vi "Grid Measurements Example - Topo & GridSpectr.vi"(6 "Internal use":string, 7 "Grid param":T1 {"height (m)" format="%#_6p"; "width (m)" format="%#_6p"; "center Y (m)" format="%#_6p"; "center X (m)" format="%#_6p"}, 8 "Error in (no error)":errorcluster, 9 "Points Y/Index Y":i32, 10 "Points X/Index X":i32, 11 "Method":enum16{"init", "run", "end"}(ring)) -> (0 "Error out":errorcluster)   [LabVIEW 2016]
doc: "Example of a measurement VI to be used in the \"Experiments on a Grid\" tool as external VI.\n\nThis example measure the topography and spectroscopy data. The spectroscopy measurements are taken on a subgrid. The data are saved to a sxm and a binary file.\n\n- Nanonis Programming Interface -"
uses:
  Nanonis Prog Interface.lvlib
  Instance           1 53Saved   Grid Measurements Example - Topo & GridSpectr .vi
panel:
  in  "Y subgrid spacing":u16=4
  in  "X subgrid spacing":u16=4
  # "Example of a measurement VI to be used in the \"Experiments on a Grid\" tool as external VI.\n\nThis example measure the topography and spectroscopy data. The spectroscopy measurements are taken on a subgrid. The data are saved to a sxm and a binary file.\n\nTo use it, set up the bias spectroscopy module to record the desired channels and set all other spectroscopy parameters. Then, set up the experiments on a grid module to use this VI as \"external VI\". On this VI's front panel, adjust the subgrid spacing.\n\n\"Experiments on a Grid\" will first (before starting the measurements) call the external VI with the \"init\" method, passing the grid resolution (Points X, Points Y) and the grid dimensions (Grid).\nThen, for the measurements, the external VI will be called with the \"run\" method, passing the current X and Y indices (Index X, Index Y).\nAfter the last measurement, the external VI will be called using the \"end\" method.\n\nSee diagram for more information about this example."
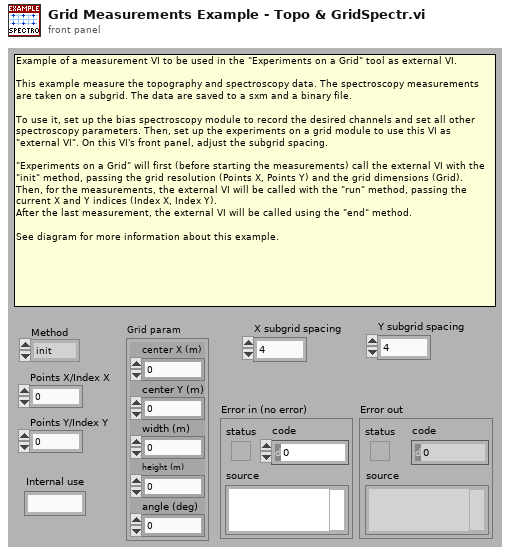
[diagram p1: front panel]
types:
  T1 = cluster{"center X (m)":sgl, "center Y (m)":sgl, "width (m)":sgl, "height (m)":sgl, "angle (deg)":sgl}
  T2 = cluster{"center X":sgl, "center Y":sgl, "angle":sgl, "width":sgl, "height":sgl, "# pixels":i32, "# lines":i32}
  T3 = cluster{"Name":string, "Calibration":sgl, "Offset":sgl, "Channel index":i32}[]
  T4 = cluster{"up/down":bool, "time/line":sgl, "start time":timestamp, "end time":timestamp}
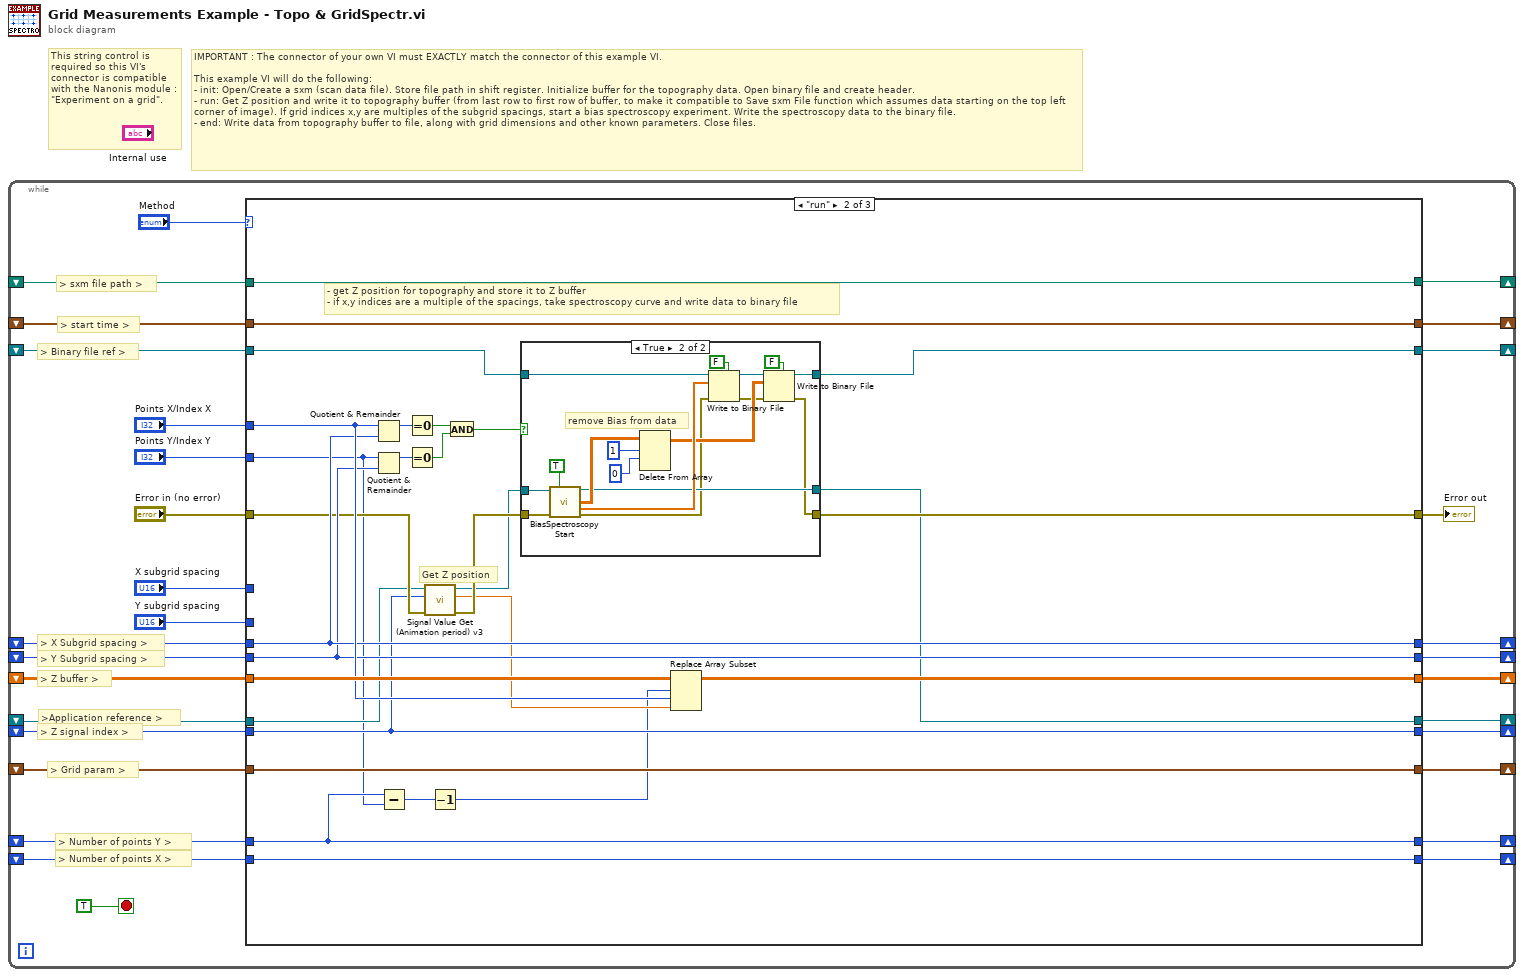
[diagram p0: block diagram]
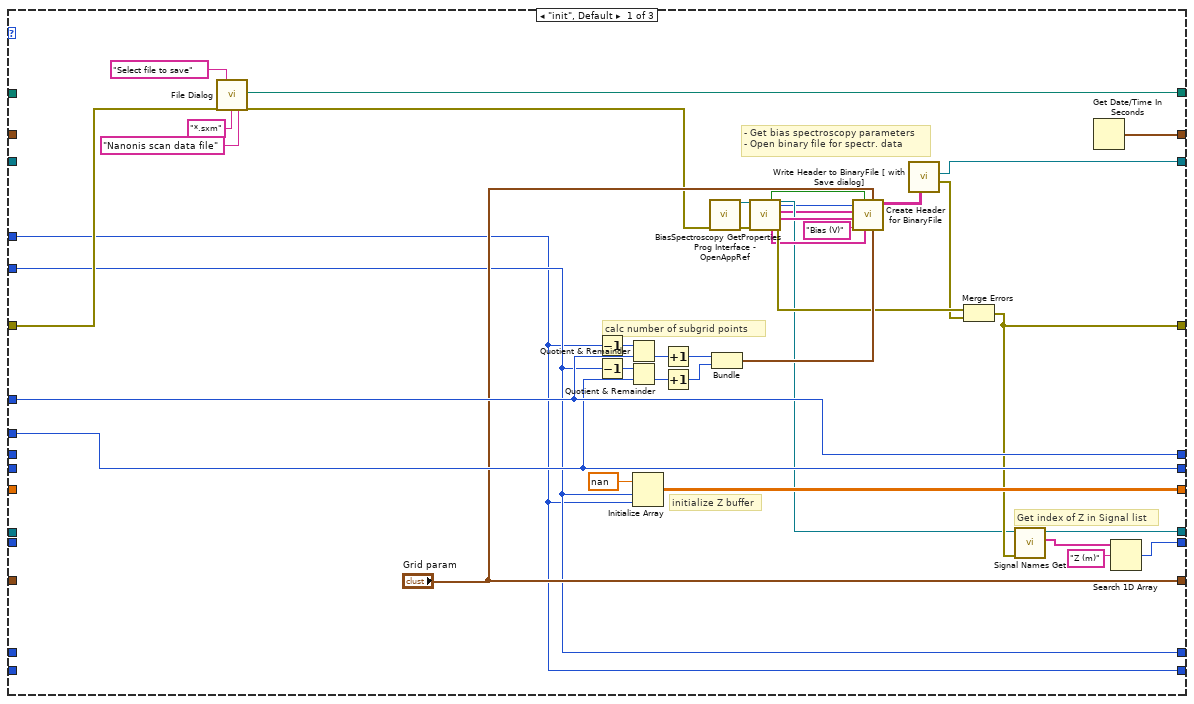
[diagram p2: hidden frame]
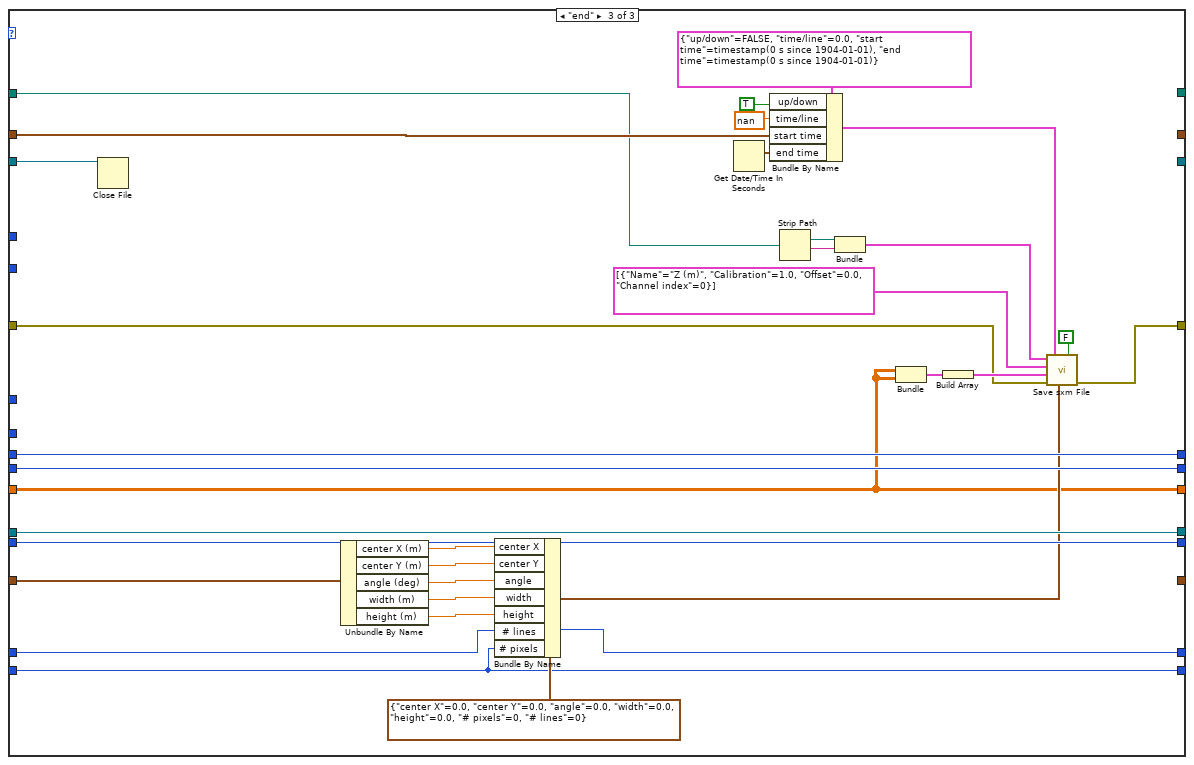
[diagram p4: hidden frame]
diagram:
  # "This string control is required so this VI's connector is compatible with the Nanonis module : \"Experiment on a grid\"."
  # "IMPORTANT : The connector of your own VI must EXACTLY match the connector of this example VI.\n\nThis example VI will do the following:\n- init: Open/Create a sxm (scan data file). Store file path in shift register. Initialize buffer for the topography data. Open binary file and create header.\n- run: Get Z position and write it to topography buffer (from last row to first row of buffer, to make it compatible to Save sxm File function which assumes data starting on the top left corner of image). If grid indices x,y are multiples of the subgrid spacings, start a bias spectroscopy experiment. Write the spectroscopy data to the binary file.\n- end: Write data from topography buffer to file, along with grid dimensions and other known parameters. Close files."
  n1 = while {
    shift-right: [w5] -> _
    shift-left: _ -> [w28]
    shift-right: [w23] -> _
    shift-left: _ -> [w22]
    shift-right: [w20] -> _
    shift-left: _ -> [w21]
    shift-right: [w19] -> _
    shift-left: _ -> [w18]
    shift-right: [w12] -> _
    shift-left: _ -> [w14]
    shift-right: [w13] -> _
    shift-left: _ -> [w15]
    shift-right: [w11] -> _
    shift-left: _ -> [w10]
    shift-right: [w9] -> _
    shift-left: _ -> [w8]
    shift-right: [w7] -> _
    shift-left: _ -> [w6]
    shift-right: [w4] -> _
    shift-left: _ -> [w3]
    shift-right: [w2] -> _
    shift-left: _ -> [w1]
    stop <- TRUE stop-if-true
    # "> Number of points X >"
    # "> Number of points Y >"
    # "> Grid param >"
    # "> start time >"
    # ">Application reference >"
    # "> Y Subgrid spacing >"
    # "> X Subgrid spacing >"
    # "> Z signal index >"
    # "> Binary file ref >"
    # "> Z buffer >"
    # "> sxm file path >"
    n2 = case shown="\"run\"" "Method" {
      tunnel: [w35 w97 _] -> w5
      tunnel: w28 -> [_ w97 w138]
      tunnel: "Error in (no error)" -> [w37 w83 w130]
      tunnel: [w47 w96 w129] -> w26
      tunnel: "Points X/Index X" -> [w31 w91 _]
      tunnel: "Points Y/Index Y" -> [w32 w72 _]
      tunnel: [w69 w94 w118] -> w23
      tunnel: w22 -> [_ w95 w118]
      tunnel: w21 -> [_ w93 w148]
      tunnel: [w60 w92 _] -> w20
      tunnel: [w58 w81 w149] -> w19
      tunnel: w18 -> [_ w81 w149]
      tunnel: "X subgrid spacing" -> [w57 _ _]
      tunnel: "Y subgrid spacing" -> [w56 _ _]
      tunnel: w15 -> [_ w85 w147]
      tunnel: w14 -> [_ w84 w146]
      tunnel: [w57 w85 w147] -> w13
      tunnel: [w56 w84 w146] -> w12
      tunnel: [w43 w77 w145] -> w11
      tunnel: w10 -> [_ w79 w145]
      tunnel: ["Grid param" w75 _] -> w9
      tunnel: w8 -> [_ w75 w128]
      tunnel: [w39 w76 _] -> w7
      tunnel: w6 -> [_ w76 w139]
      tunnel: [w32 w73 w119] -> w4
      tunnel: w3 -> [_ w73 w119]
      tunnel: [w31 w74 w120] -> w2
      tunnel: w1 -> [_ w74 w120]
      frame "init", Default {
        # "- Get bias spectroscopy parameters\n- Open binary file for spectr. data"
        # "initialize Z buffer"
        # "calc number of subgrid points"
        # "Get index of Z in Signal list"
        n3 = call "File Dialog"("prompt"="Select file to save", "error in"=w37, "pattern (all files)"="*.sxm" ("pattern"), "pattern label"="Nanonis scan data file") -> ("selected path"=w35:path, "error out"=w36:errorcluster)  [unwired: 8 in, 2 out]
        n4 = Decrement(x=w31) -> (x-1=w55:i32)
        n5 = Decrement(x=w32) -> (x-1=w54:i32)
        n6 = Quotient & Remainder(x=w55, y=w57) -> (floor(x/y)=w53:i32)  [unwired: 1 out]
        n7 = Quotient & Remainder(x=w54, y=w56) -> (floor(x/y)=w52:i32)  [unwired: 1 out]
        n8 = Initialize Array(sgl nan ("element"), w32, w31) -> (w69:sgl[][])
        n9 = Increment(x=w53) -> (x+1=w51:i32)
        n10 = Increment(x=w52) -> (x+1=w50:i32)
        n11 = call <userlib>:"Prog Interface - OpenAppRef.vi"("Error in (no error)"=w36) -> ("Error out"=w48:errorcluster, "Application reference"=w46:refnum<vi>)  [unwired: 5 in]
        n12 = Bundle(w51, w50) -> (w64:cluster{i32, i32})  [unwired: 1 in]
        n13 = call <userlib>:"BiasSpectroscopy GetProperties.vi"("Application ref in"=w46, "Error in (no error)"=w48) -> ("Backward sweep"=w65:bool, "Application ref out"=w45:refnum<vi>, "Number of points"=w42:i32, "Channels"=w41:string[], "Parameters"=w63:string[], "Fixed parameters"=w49:string[], "Error out"=w62:errorcluster)  [unwired: 6 in, 1 out]
        n14 = call <userlib>:"Create Header for BinaryFile.vi"("Grid points"=w64, "Grid param"="Grid param", "Fixed parameters"=w49, "Backward sweep"=w65, "Sweep signal"="Bias (V)" ("Sweep Signal"), "Parameters"=w63, "Channels"=w41, "Points per sweep"=w42) -> ("Header (fixed attributes)"=w67:string[][])  [unwired: 3 in]
        n15 = call <userlib>:"Write Header to BinaryFile [ with Save dialog].vi"("Fixed Attributes"=w67) -> ("Error out"=w61:errorcluster, "File ref"=w60:refnum<file>)  [unwired: 7 in, 2 out]
        n16 = Merge Errors(w62, w61) -> (w47:errorcluster)
        n17 = call <userlib>:"Signal Names Get.vi"("error in (no error)"=w47, "Application ref in"=w45) -> ("Signals Names"=w44:string[], "Application ref out"=w43:refnum<vi>)  [unwired: 5 in, 1 out]
        n18 = Get Date/Time In Seconds() -> (seconds since 1Jan1904=w39:timestamp)
        n19 = Search 1D Array(1D array=w44, element="Z (m)") -> (index of element=w58:i32)  [unwired: 1 in]
      }
      frame "run" {
        # "Get Z position"
        # "- get Z position for topography and store it to Z buffer\n- if x,y indices are a multiple of the spacings, take spectroscopy curve and write data to binary file"
        n20 = Quotient & Remainder(x=w91, y=w85) -> (x-y*floor(x/y)=w90:i32)  [unwired: 1 out]
        n21 = Quotient & Remainder(x=w72, y=w84) -> (x-y*floor(x/y)=w89:i32)  [unwired: 1 out]
        n22 = Subtract(x=w73, y=w72) -> (x-y=w71:i32)
        n23 = Equal To 0?(x=w90) -> (x = 0?=w88:bool)
        n24 = Equal To 0?(x=w89) -> (x = 0?=w87:bool)
        n25 = call <userlib>:"Signal Value Get (Animation period) v3.vi"("error in (no error)"=w83, "Signal index (0-127)"=w81, "Application ref in"=w79) -> ("error out"=w82:errorcluster, "Signal value"=w80:sgl, "Application ref out"=w78:refnum<vi>)  [unwired: 5 in]
        n26 = Decrement(x=w71) -> (x-1=w70:i32)
        n27 = And(x=w88, y=w87) -> (x .and. y?=w86:bool)
        n28 = case shown="True" w86 {
          tunnel: [w99 w101] -> w96
          tunnel: w93 -> [w100 w117]
          tunnel: [w100 w115] -> w92
          tunnel: w82 -> [w99 w114]
          tunnel: w78 -> [w98 w106]
          tunnel: [w98 w105] -> w77
          frame False {
            # "Point indices aren't multiple of subgrid spacing\n=> no spectroscopy at this point"
          }
          frame True {
            # "remove Bias from data"
            n29 = call <userlib>:"BiasSpectroscopy Start.vi"("Application ref in"=w106, "Get data (F)"=TRUE ("Get Data (F)"), "Error in (no error)"=w114) -> ("Application ref out"=w105:refnum<vi>, "Data"=w113:sgl[][], "Parameters"=w112:sgl[], "Error out"=w103:errorcluster)  [unwired: 8 in, 1 out]
            n30 = Delete From Array(array=w113, length=1, index (row)=0 ("index")) -> (array with subset deleted=w111:sgl[][])  [unwired: 1 in, 1 out]
            n31 = Write to Binary File(file (use dialog)=w117, data=w112, error in=w103, 5:FALSE ("prepend array or string size? (T)")) -> (refnum out=w116:refnum<file>, error out=w102:errorcluster)  [unwired: 2 in, 1 out]
            n32 = Write to Binary File(file (use dialog)=w116, data=w111, error in=w102, 5:FALSE ("prepend array or string size? (T)")) -> (refnum out=w115:refnum<file>, error out=w101:errorcluster)  [unwired: 2 in, 1 out]
          }
        }
        n33 = Replace Array Subset(array=w95, new element=w80, index (row)=w70, index (col)=w91) -> (w94:sgl[][])
      }
      frame "end" {
        n34 = Close File(refnum=w148) -> ()  [unwired: 1 in, 2 out]
        n35 = Unbundle By Name(w128) -> ("center X (m)"=w126:sgl, "center Y (m)"=w125:sgl, "angle (deg)"=w124:sgl, "width (m)"=w123:sgl, "height (m)"=w122:sgl)
        n36 = Bundle By Name(cluster=T2 {"center X"=0.0, "center Y"=0.0, "angle"=0.0, "width"=0.0, "height"=0.0, "# pixels"=0, "# lines"=0} ("Scanfield"), "center X"=w126, "center Y"=w125, "angle"=w124, "width"=w123, "height"=w122, "# lines"=w119, "# pixels"=w120) -> (w121:T2)
        n37 = Get Date/Time In Seconds() -> (seconds since 1Jan1904=w136:timestamp)
        n38 = Bundle By Name(cluster=T4 {"up/down"=FALSE, "time/line"=0.0, "start time"=timestamp(0 s since 1904-01-01), "end time"=timestamp(0 s since 1904-01-01)} ("Scan param"), "up/down"=TRUE, "time/line"=sgl nan ("input 7"), "start time"=w139, "end time"=w136) -> (w137:T4)
        n39 = Strip Path(path=w138) -> (stripped path=w133:path, name=w132:string)
        n40 = Bundle("stripped path"=w133, "name"=w132) -> (w131:cluster{"stripped path":path, "name":string})  [unwired: 1 in]
        n41 = Bundle(w118, w118) -> (w144:cluster{sgl[][], sgl[][]})  [unwired: 1 in]
        n42 = Build Array(w144) -> (w143:cluster{sgl[][], sgl[][]}[])
        n43 = call "Save sxm File.vi"("Auto file naming? (T)"=FALSE, "Scanfield"=w121, "Scan param"=w137, "error in (no error)"=w130, "Channels data"=w143, "Channels config"=T3 [{"Name"="Z (m)", "Calibration"=1.0, "Offset"=0.0, "Channel index"=0}], "Filename control"=w131) -> ("error out"=w129:errorcluster)  [unwired: 2 in, 2 out]
      }
    }
    "Error out" <- w26
  }
